vi "destroy.vi"(8 "error in (no error)":errorcluster, 11 "Camera Controller in":refnum<class "Camera Controller.lvclass">) -> (0 "error out":errorcluster, 3 "Camera Controller out":refnum<class "Camera Controller.lvclass">)   [LabVIEW 2022 SP3, in "Camera Controller.lvclass"]
uses:
  Camera Controller.lvclass
  Camera Controller.lvclass/Camera Controller.ctl
  XY Stage/Process Actor/Process Framework/Interlock Q Class/Interlock Q Class.lvclass
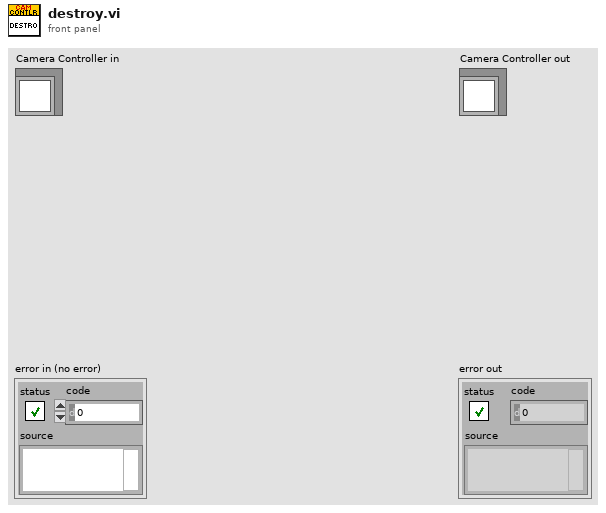
[diagram p1: front panel]
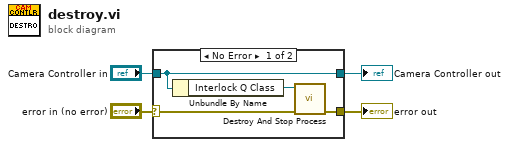
[diagram p0: block diagram]
diagram:
  n1 = case shown="No Error" "error in (no error)" {
    selector: "error in (no error)" -> [w6 w10]
    tunnel: [w5 w10] -> w3
    tunnel: [w8 w9] -> w1
    tunnel: "Camera Controller in" -> [w8 w9]
    frame No Error {
      n2 = Unbundle By Name(w8) -> ("Interlock Q Class"=w7:refnum<class "Interlock Q Class.lvclass">)
      n3 = call-dynamic "Destroy And Stop Process.vi"("error in (no error)"=w6, "Interlock Q Class in"=w7) -> ("error out"=w5:errorcluster)  [unwired: 8 in, 1 out]
    }
    frame Error {
    }
  }
  "error out" <- w3
  "Camera Controller out" <- w1
